vi "PE Get Wavelength Range.vi"(8 "error in (no error)":errorcluster, 11 "peHandle":u32) -> (0 "error out":errorcluster, 1 "function return":i32, 2 "maximum":dbl, 3 "minimum":dbl)   [LabVIEW 2011, in "libPhyspec.lvlib"]
doc: "PHYSPEC_API PE_STATUS PE_GetWavelengthRange(CPE_HANDLE peHandle, double *minimum, double *maximum);"
uses:
  libPhyspec.lvlib
  libPhyspec.dll
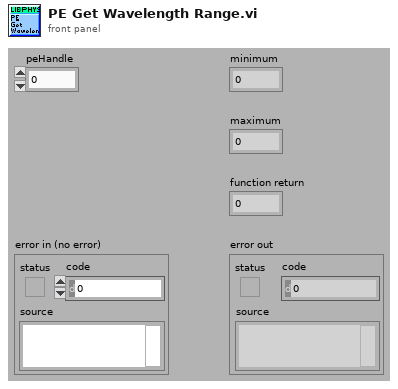
[diagram p1: front panel]
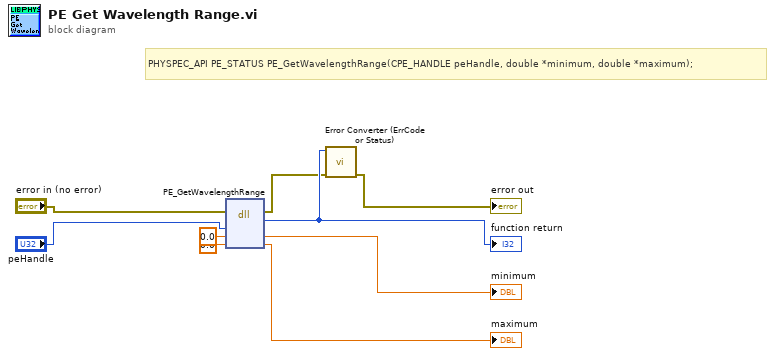
[diagram p0: block diagram]
diagram:
  # "PHYSPEC_API PE_STATUS PE_GetWavelengthRange(CPE_HANDLE peHandle, double *minimum, double *maximum);"
  n1 = dll-call lib="D:/users/nicolas/PHySpec-SDK-1.0.0/Labview-example/libPhyspec/libPhyspec.*" fn="PE_GetWavelengthRange"(error in="error in (no error)", "peHandle"="peHandle", "minimum"=0.0, "maximum"=0.0) -> (error out=w2:errorcluster, w9:i32, "minimum"=→"minimum":dbl, "maximum"=→"maximum":dbl)  [unwired: 3 in, 1 out]
  "function return" <- w9
  n2 = call "Error Converter (ErrCode or Status).vi"("error in (no error)"=w2, "error code"=w9) -> ("error out"=→"error out":errorcluster)  [unwired: 9 in]
